vi "Mod_OFDM_Get_OFDM_Symbol_Pool.vi"(0 "Configuration in":variant, 1 "Symbol Pool":u16, 11 "error in":errorcluster) -> (2 "Symbol Status":bool, 4 "Configuration out":variant, 6 "Attribute Name":string, 8 "Symbol Pool":string[](array[string]), 14 "Symbol Pool":u16, 15 "error out":errorcluster)   [LabVIEW 2010]
doc: "The VI retrives the attribute containing information about the OFDM symbols that have been configured. This is an array of strings, where each element represents teh name of the OFDM Symbol. These names may be used to retrieve the information about the respective OFDM symbol."
uses:
  Controls(Type_DEf)/Attribute Data Types.ctl
  Controls(Type_DEf)/Configure Pulse Shaping.ctl
  Controls(Type_DEf)/Pool of Modulator Control.ctl
  Controls(Type_DEf)/Pool of Data Source Control.ctl
  Controls(Type_DEf)/Attribute Names.ctl
panel:
  in  "Attribute Data Types":T1={"Pulse Shaping"={"System Filter"={"TX Filter"=enum."none", "Alpha"=0.0, "filter length"=0}, "Modulation system parameters"={"samples per symbol (16)"=0}, "symbol rate (Hz)"=0.0}, "FRAME Table"=[], "OFDM Frame"=[], "Sub Carrier Selection"={"Sub Carrier Selection"=[], "OFDM Parameters"={"# of Sub Carrier"=0, "Length Of Cylic Prefix"=0}}, "Symbol Table"=[], "Symbol Pool"=[], "Pool of Modulators"=[], "Pool of Data Sources"=[], "Atribute Names"={"Data Source Pool"="Data Source Pool ", "Modulator Source Pool"="Modulator Source Pool ", "OFDM SYMBOL POOL"="OFDM SYMBOL POOL", "Symbol Table"="Symbol Table", "Sub Carrier Selection"="Sub Carrier Selection", "OFDM Frame"="OFDM Frame", "FRAME Table"="FRAME Table", "Pulse Shaping"="Pulse Shaping"}} {"Pool of Data Sources"."Register Initial State" format="%08x"; "Pulse Shaping"."symbol rate (Hz)" min=1.0 step=1.0 format="%.2p"; "Pulse Shaping"."Modulation system parameters"."samples per symbol (16)" step=2; "Pulse Shaping"."System Filter"."Alpha" min=0.0 max=1.0 step=0.05 format="%.2f"}
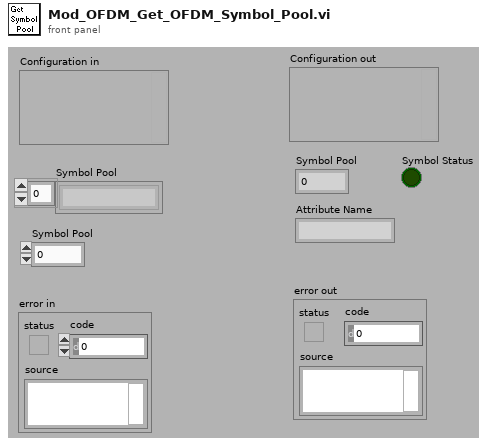
[diagram p1: front panel]
types:
  T1 = typedef "Attribute Data Types.ctl" = cluster{"Pulse Shaping":T2, "FRAME Table":string[][], "OFDM Frame":cluster{"Symbol Name":string, "# of Symbols":i32}[], "Sub Carrier Selection":cluster{"Sub Carrier Selection":cluster{"Sub Carrier":bool, "Data Source":u16, "Modulator":u16}[], "OFDM Parameters":cluster{"# of Sub Carrier":i32, "Length Of Cylic Prefix":i32}}, "Symbol Table":string[][], "Symbol Pool":string[], "Pool of Modulators":T3, "Pool of Data Sources":T4, "Atribute Names":T5}
  T2 = typedef "Configure Pulse Shaping.ctl" = cluster{"System Filter":cluster{"TX Filter":enum16{"none", "Raised Cosine", "Root Raised Cos"}, "Alpha":dbl, "filter length":i32}, "Modulation system parameters":cluster{"samples per symbol (16)":u32}, "symbol rate (Hz)":dbl}
  T3 = typedef "Pool of Modulator Control.ctl" = cluster{"M-QAM":enum16{"4", "16", "64", "256"}, "M-PSK":enum16{"2", "4", "8", "16", "32", "64", "128", "256"}, "Type of Modulation":enum16{"PSK", "QAM"}, " PSK":cluster{"differential PSK":enum16{"disable", "enable"}, "PSK type":enum16{"normal", "shifted", "offset"}}}[]
  T4 = typedef "Pool of Data Source Control.ctl" = cluster{"mode (PN)":enum16{"PN", "pattern", "user"}, "PN sequence order (9)":i32, "Invert Output Bits":enum16{"No", "Yes"}, "Register Initial State ":u32, "User base bit pattern":i8[], "base bit pattern (00001111)":enum16{"0", "1", "01", "0011", "00001111"}, "Reset to Initial State":enum16{"Every OFDM Frame", "Every OFDM Symbol", "Every Sub Carrier"}}[]
  T5 = typedef "Attribute Names.ctl" = cluster{"Data Source Pool":string, "Modulator Source Pool":string, "OFDM SYMBOL POOL":string, "Symbol Table":string, "Sub Carrier Selection":string, "OFDM Frame":string, "FRAME Table":string, "Pulse Shaping":string}
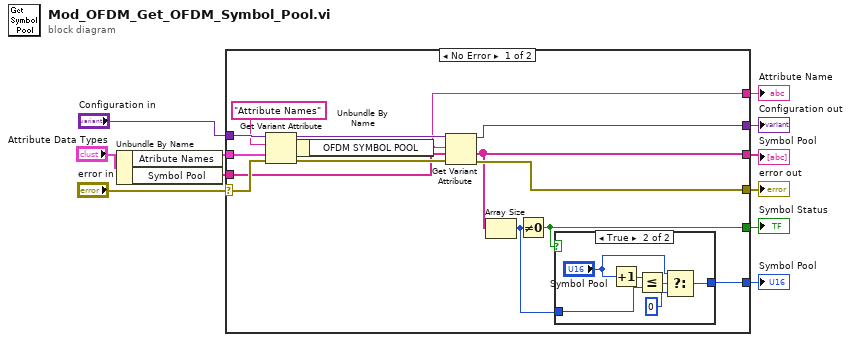
[diagram p0: block diagram]
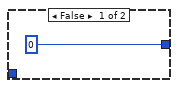
[diagram p2: hidden frame]
diagram:
  n1 = Unbundle By Name("Attribute Data Types") -> ("Atribute Names"=w6:T5, "Symbol Pool"=w5:string[])
  n2 = case shown="No Error" "error in" {
    selector: "error in" -> [w22 w34]
    tunnel: [w26 w34] -> w10
    tunnel: "Configuration in" -> [w24 _]
    tunnel: [w25 _] -> w8
    tunnel: w6 -> [w18 _]
    tunnel: w5 -> [w20 _]
    tunnel: [w15 _] -> w4
    tunnel: [w16 _] -> w3
    tunnel: [w14 _] -> w2
    tunnel: [w13 _] -> w1
    frame No Error {
      n3 = Get Variant Attribute(Variant=w24, name="Attribute Names", default value (empty Variant)=w18, error in=w22) -> (duplicate Variant=w23:variant, value=w17:T5, error out=w21:errorcluster)  [unwired: 1 out]
      n4 = Unbundle By Name(w17) -> ("OFDM SYMBOL POOL"=w16:string)
      n5 = Get Variant Attribute(Variant=w23, name=w16, default value (empty Variant)=w20, error in=w21) -> (duplicate Variant=w25:variant, value=w15:string[], error out=w26:errorcluster)  [unwired: 1 out]
      n6 = Array Size(array=w15) -> (size(s)=w12:i32)
      n7 = Not Equal To 0?(x=w12) -> (x != 0?=w14:bool)
      n8 = case shown="True" w14 {
        tunnel: [u16 0 ("Symbol Pool") w29] -> w13
        tunnel: w12 -> [_ w33]
        frame False {
        }
        frame True {
          n9 = Increment(x="Symbol Pool") -> (x+1=w31:u16)
          n10 = Less Or Equal?(x=w31, y=w33) -> (x <= y?=w32:bool)
          n11 = Select(t="Symbol Pool", s=w32, f=u16 0) -> (s? t:f=w29:u16)
        }
      }
    }
    frame Error {
    }
  }
  "error out" <- w10
  "Configuration out" <- w8
  "Symbol Pool" <- w4
  "Attribute Name" <- w3
  "Symbol Status" <- w2
  "Symbol Pool" <- w1
